vi "Loop_CalculateDegree (SubVI).vi"() -> ()   [LabVIEW 2017]
panel:
  out "Output Position":dbl
  in  "Desired Degree":dbl
  in  "Max Encoder Ticks (1 Rotation)":dbl format="%#_13g"
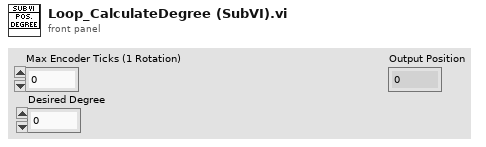
[diagram p1: front panel]
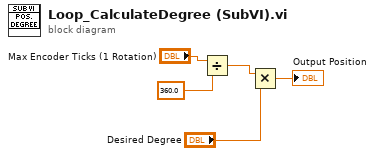
[diagram p0: block diagram]
diagram:
  n1 = Divide(x="Max Encoder Ticks (1 Rotation)", y=360.0) -> (x/y=w3:dbl)
  n2 = Multiply(x=w3, y="Desired Degree") -> (x*y=→"Output Position":dbl)
